vi "x-axis.vi"(8 "error in (no error)":errorcluster, 11 "Magnetic Field Lakeshore Continuous in":refnum<class "Magnetic Field Lakeshore Continuous.lvclass">) -> (0 "error out":errorcluster, 1 "Label":string, 2 "Unit":string, 3 "Magnetic Field Lakeshore Continuous out":refnum<class "Magnetic Field Lakeshore Continuous.lvclass">)   [LabVIEW 2023, in "Magnetic Field Lakeshore Continuous.lvclass"]
uses:
  Magnetic Field Lakeshore Continuous.lvclass
  Scanner/Scanner.lvclass
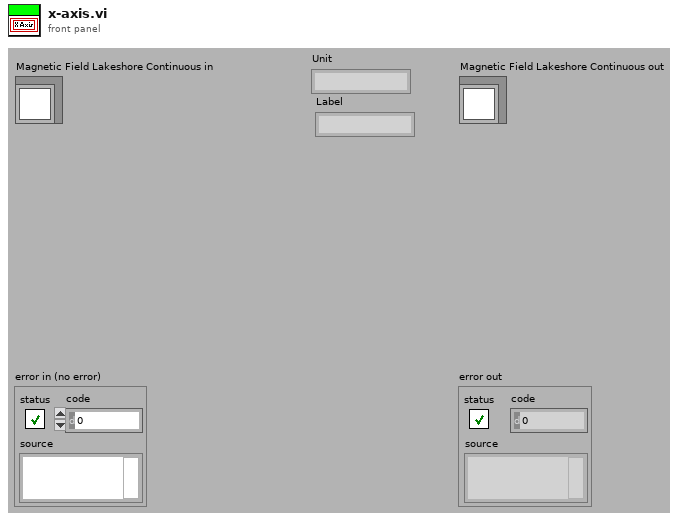
[diagram p1: front panel]
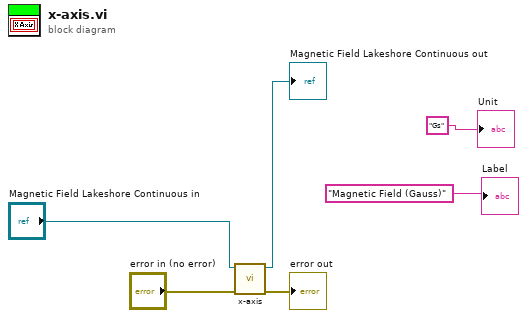
[diagram p0: block diagram]
diagram:
  n1 = call-parent "x-axis.vi"("error in (no error)"="error in (no error)", "Scanner in"="Magnetic Field Lakeshore Continuous in") -> ("error out"=→"error out":errorcluster, "Scanner out"=→"Magnetic Field Lakeshore Continuous out":refnum<class "Magnetic Field Lakeshore Continuous.lvclass">)  [unwired: 6 in, 2 out]
  "Label" <- "Magnetic Field (Gauss)" ("Label")
  "Unit" <- "Gs" ("Unit")
